vi "appendXMLOntrak.vi"(8 "Ontrak Channel":i32, 9 "error in (no error)":errorcluster, 10 "Parent Camera Node":refnum<k20>, 11 "DOM document in":refnum<k20>) -> (0 "error out":errorcluster)   [LabVIEW 2013]
uses:
  <resource>/objmgr/DOMUserDefRef.rc
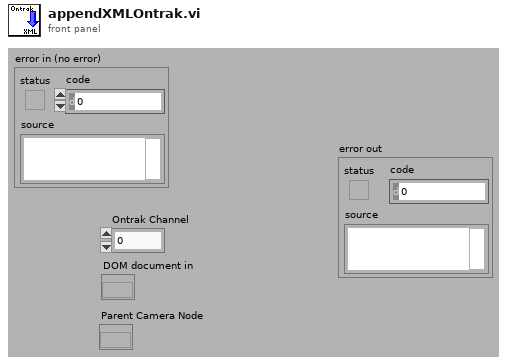
[diagram p1: front panel]
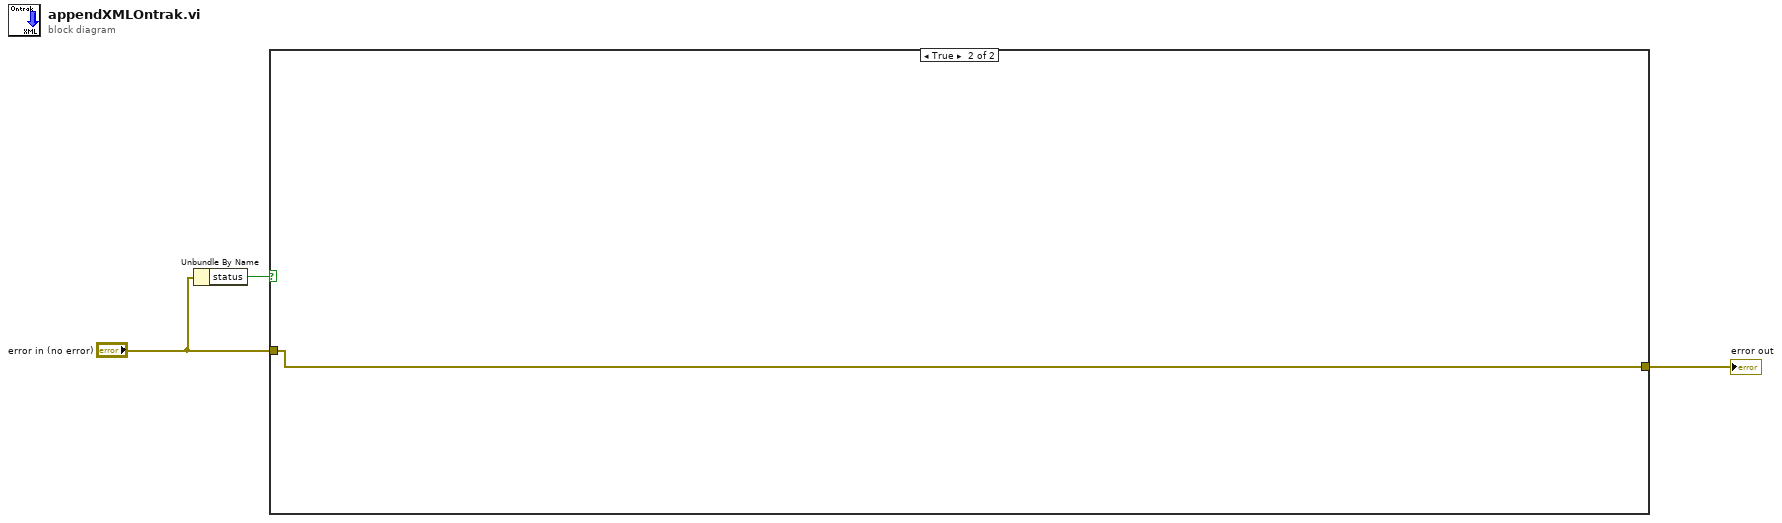
[diagram p0: block diagram]
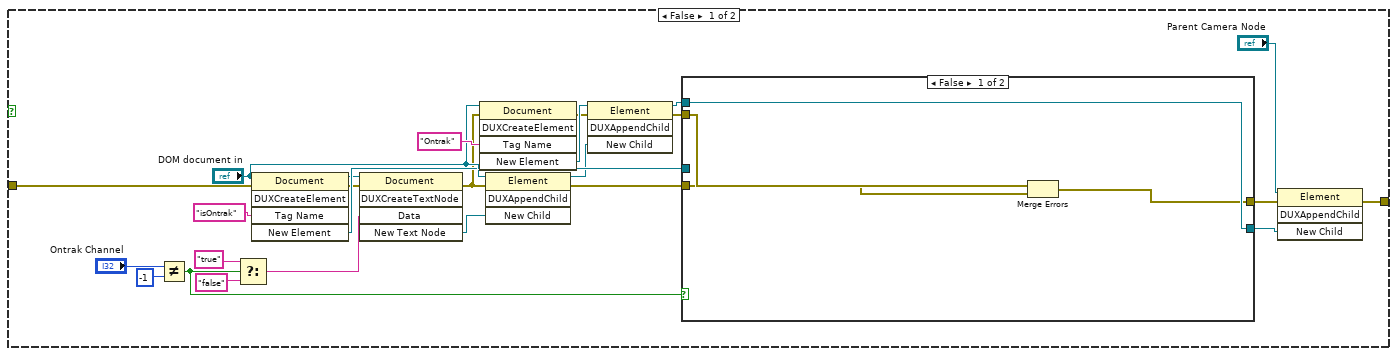
[diagram p2: hidden frame]
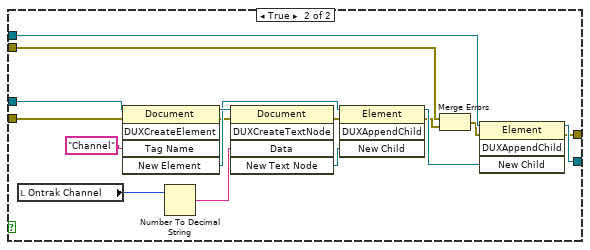
[diagram p3: hidden frame]
diagram:
  n1 = Unbundle By Name("error in (no error)") -> ("status"=w2:bool)
  n2 = case shown="True" w2 {
    tunnel: "error in (no error)" -> [w5 w50]
    tunnel: [w4 w50] -> w3
    frame False {
      n3 = Not Equal?(x="Ontrak Channel", y=-1) -> (x != y?=w14:bool)
      n4 = Select(t="true", s=w14, f="false") -> (s? t:f=w15:string)
      n5 = invoke class="Document" method="DUXCreateElement"(reference="DOM document in", error in=w5, "Tag Name"="isOntrak") -> (reference out=w19:refnum<k20>, error out=w11:errorcluster, "New Element"=w20:refnum<k20>)  [unwired: 2 in, 2 out]
      n6 = invoke class="Document" method="DUXCreateTextNode"(reference=w19, error in=w11, "Data"=w15) -> (error out=w10:errorcluster, "New Text Node"=w21:refnum<k20>)  [unwired: 2 in, 3 out]
      n7 = invoke class="Document" method="DUXCreateElement"(reference="DOM document in", error in=w10, "Tag Name"="Ontrak") -> (error out=w9:errorcluster, "New Element"=w27:refnum<k20>)  [unwired: 2 in, 3 out]
      n8 = invoke class="Element" method="DUXAppendChild"(reference=w20, error in=w10, "New Child"=w21) -> (reference out=w18:refnum<k20>, error out=w7:errorcluster)  [unwired: 1 in, 2 out]
      n9 = invoke class="Element" method="DUXAppendChild"(reference=w27, error in=w9, "New Child"=w18) -> (reference out=w13:refnum<k20>, error out=w8:errorcluster)  [unwired: 1 in, 2 out]
      n10 = case shown="False" w14 {
        tunnel: "DOM document in" -> [_ w48]
        tunnel: w13 -> [w32 w41]
        tunnel: [w32 w40] -> w12
        tunnel: w8 -> [w31 w35]
        tunnel: w7 -> [w30 w39]
        tunnel: [w29 w33] -> w6
        frame False {
          n11 = Merge Errors(w31, w30) -> (w29:errorcluster)
        }
        frame True {
          n12 = local read "Ontrak Channel"() -> (w47:i32)
          n13 = invoke class="Document" method="DUXCreateElement"(reference=w48, error in=w39, "Tag Name"="Channel") -> (reference out=w44:refnum<k20>, error out=w38:errorcluster, "New Element"=w43:refnum<k20>)  [unwired: 2 in, 2 out]
          n14 = Number To Decimal String(number=w47) -> (decimal integer string=w45:string)  [unwired: 1 in]
          n15 = invoke class="Document" method="DUXCreateTextNode"(reference=w44, error in=w38, "Data"=w45) -> (error out=w37:errorcluster, "New Text Node"=w46:refnum<k20>)  [unwired: 2 in, 3 out]
          n16 = invoke class="Element" method="DUXAppendChild"(reference=w43, error in=w37, "New Child"=w46) -> (reference out=w42:refnum<k20>, error out=w36:errorcluster)  [unwired: 1 in, 2 out]
          n17 = Merge Errors(w35, w36) -> (w34:errorcluster)
          n18 = invoke class="Element" method="DUXAppendChild"(reference=w41, error in=w34, "New Child"=w42) -> (reference out=w40:refnum<k20>, error out=w33:errorcluster)  [unwired: 1 in, 2 out]
        }
      }
      n19 = invoke class="Element" method="DUXAppendChild"(reference="Parent Camera Node", error in=w6, "New Child"=w12) -> (error out=w4:errorcluster)  [unwired: 1 in, 3 out]
    }
    frame True {
    }
  }
  "error out" <- w3
